vi "Spectrum.vi"(0 "waveforms":waveform(dbl)[](array[waveform]), 5 "maximum harmonic order (50)":u16=50, 9 "system info in":refnum<class "EP System Info.lvclass">, 11 "error in (no error)":errorcluster) -> (4 "spectra":T2(array[cluster]), 10 "system info out":refnum<class "EP System Info.lvclass">, 15 "error out":errorcluster)   [LabVIEW 2014, in "NI_EP_Power Quality.lvlib"]
doc: "Calculates the fast Fourier transform (FFT) spectra from voltage signals, current signals, or signals that contain both voltage and current. This VI returns FFT spectra as complex spectra up to <B>maximum harmonic order</B> with a frequency resolution around 5 Hz. The frequency resolution is the fundamental frequency divided by 10 or 12.\n\nThis VI supports measuring single-line and multiple-line systems."
uses:
  <vilib>/addons/Electrical Power/PQ/NI_EP_Power Quality.lvlib
  <vilib>/addons/Electrical Power/PQ/Common/Controls/ep_AI Data Channel.ctl
  <vilib>/addons/Electrical Power/PQ/Common/Classes/System Info/EP System Info.lvclass
  <vilib>/addons/Electrical Power/Power Measurement/NI_EP_Power Measurement.lvlib
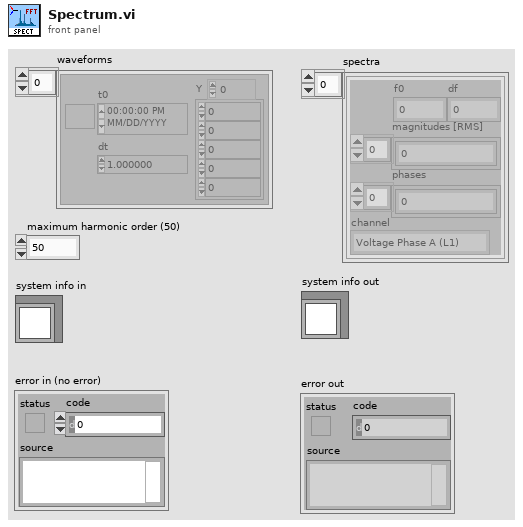
[diagram p1: front panel]
types:
  T1 = typedef "NI_EP_Power Quality.lvlib/ep_AI Data Channel.ctl" = enum16{"Voltage Phase A (L1)", "Voltage Phase B (L2)", "Voltage Phase C (L3)", "Voltage Phase N (Neutral)", "Current Phase A (L1)", "Current Phase B (L2)", "Current Phase C (L3)", "Current Phase N (Neutral)"}
  T2 = cluster{"f0":dbl, "df":dbl, "magnitudes [RMS]":dbl[], "phases":dbl[], "channel":T1}[]
  T3 = cluster{"f0":dbl, "df":dbl, "magnitude":dbl[], "phase":dbl[], "channel":T1}
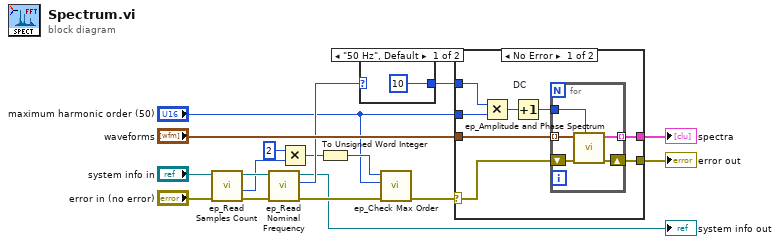
[diagram p0: block diagram]
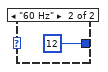
[diagram p2: hidden frame]
diagram:
  n1 = call <vilib>:"ep_Read Samples Count.vi"("error in (no error)"="error in (no error)", "system info in"="system info in") -> ("error out"=w11:errorcluster, "half-cycle (samples)"=w8:i32, "system info out"=w12:refnum<class "EP System Info.lvclass">)  [unwired: 5 in, 2 out]
  n2 = call <vilib>:"ep_Read Nominal Frequency.vi"("error in (no error)"=w11, "system info in"=w12) -> ("error out"=w5:errorcluster, "nominal frequency"=w10:enum16{"50 Hz", "60 Hz"}, "system info out"=→"system info out":refnum<class "EP System Info.lvclass">)  [unwired: 6 in, 1 out]
  n3 = Multiply(x=2, y=w8) -> (x*y=w6:i32)
  n4 = To Unsigned Word Integer(number=w6) -> (unsigned 16bit integer=w3:u16)
  n5 = case shown="\"50 Hz\", Default" w10 {
    tunnel: [u16 10 u16 12] -> w9
    frame "50 Hz", Default {
    }
    frame "60 Hz" {
    }
  }
  n6 = call <vilib>:"ep_Check Max Order.vi"("error in (no error)"=w5, "maximum harmonic order"="maximum harmonic order (50)", "samples per cycle"=w3) -> ("error out"=w4:errorcluster)  [unwired: 8 in]
  n7 = case shown="No Error" w4 {
    selector: w4 -> [w21 w33]
    tunnel: "waveforms" -> [w27 _]
    tunnel: [w20 w33] -> w16
    tunnel: [w26 _] -> w15
    tunnel: "maximum harmonic order (50)" -> [w25 _]
    tunnel: w9 -> [w22 _]
    frame No Error {
      n8 = Multiply(x=w22, y=w25) -> (x*y=w24:u16)
      n9 = Increment "DC"(x=w24) -> (x+1=w23:u16)
      n10 = for {
        tunnel: w27 -> [w30] mode=indexing
        tunnel: w23 -> [w32]
        tunnel: [w31] -> w26 mode=indexing
        shift-right: [w28] -> w20
        shift-left: w21 -> [w29]
        n11 = call <vilib>:"ep_Amplitude and Phase Spectrum.vi"("# of bins"=w32, "error in (no error)"=w29, "waveform"=w30) -> ("error out"=w28:errorcluster, "spectrum"=w31:T3)  [unwired: 7 in]
      }
    }
    frame Error {
    }
  }
  "error out" <- w16
  "spectra" <- w15
